vi "Check-Temperature-value-settings.vi"(8 "error in":errorcluster, 9 "Correct. params. ref.":refnum<data-value>, 10 "Config. params. ref.":refnum<data-value>, 11 "Temp. params. ref.":refnum<data-value>) -> (0 "error IO":errorcluster, 3 "Passed?":bool)   [LabVIEW 2013, in "CameraVision.lvlib" / "CV-Temperature.lvclass"]
uses:
  CV-Temperature.lvclass
  Configuration/CV-Configuration.lvclass
  Correction/CV-Correction.lvclass
  CV-Temperature.lvclass/CV-Temperature.ctl
  Configuration/CV-Configuration.lvclass/CV-Configuration.ctl
  Correction/CV-Correction.lvclass/CV-Correction.ctl
  Read Temperature value.vi
  Read Temperature field.vi
  Configuration/Read Number of cameras.vi
  Correction/Read 2nd image correlation.vi
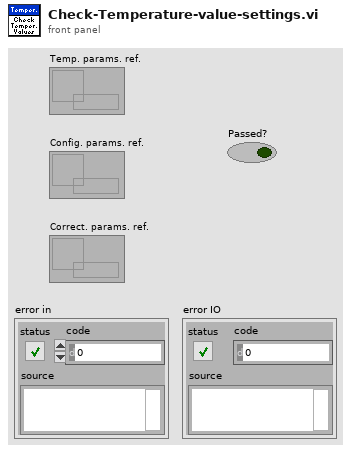
[diagram p1: front panel]
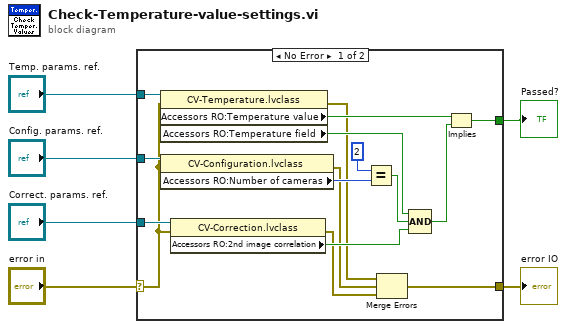
[diagram p0: block diagram]
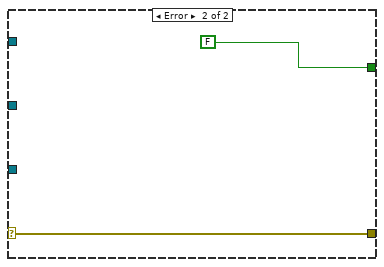
[diagram p2: hidden frame]
diagram:
  n1 = case shown="No Error" "error in" {
    selector: "error in" -> [w7 w23]
    tunnel: "Correct. params. ref." -> [w13 _]
    tunnel: [w8 w23] -> w5
    tunnel: [w21 FALSE] -> w6
    tunnel: "Temp. params. ref." -> [w20 _]
    tunnel: "Config. params. ref." -> [w18 _]
    frame No Error {
      n2 = property class="CV-Temperature.lvclass"(reference=w20, error in=w7) -> (error out=w11:errorcluster, "Accessors RO:Temperature value"=w19:bool, "Accessors RO:Temperature field"=w16:bool)  [unwired: 1 out]
      n3 = property class="CV-Configuration.lvclass"(reference=w18, error in=w7) -> (error out=w10:errorcluster, "Accessors RO:Number of cameras"=w15:i32)  [unwired: 1 out]
      n4 = property class="CV-Correction.lvclass"(reference=w13, error in=w7) -> (error out=w9:errorcluster, "Accessors RO:2nd image correlation"=w12:bool)  [unwired: 1 out]
      n5 = Equal?(x=2 ("y"), y=w15) -> (x = y?=w17:bool)
      n6 = Merge Errors(w11, w10, w9) -> (w8:errorcluster)
      n7 = Compound Arithmetic op=AND(w16, w17, w12) -> (w22:bool)
      n8 = Implies(1:w22, 2:w19) -> (0:w21:bool)
    }
    frame Error {
    }
  }
  "Passed?" <- w6
  "error IO" <- w5
